vi "Read JsonContent.vi"(8 "error in (no error)":errorcluster, 11 "object in":refnum<class "TAFConfiguration.lvclass">) -> (0 "error out":errorcluster, 2 "JsonContent":string, 3 "object out":refnum<class "TAFConfiguration.lvclass">)   [LabVIEW 2021, in "TAF Proj Document Type.lvlib" / "TAFConfiguration.lvclass"]
uses:
  <vilib>/Wovalab/AntiDoc/Document Type/Add-ons/LabVIEW TAF Project/TAFConfiguration/TAFConfiguration.lvclass
  <vilib>/Wovalab/AntiDoc/Document Type/Add-ons/LabVIEW TAF Project/TAFConfiguration/TAFConfiguration.lvclass/TAFConfiguration.ctl
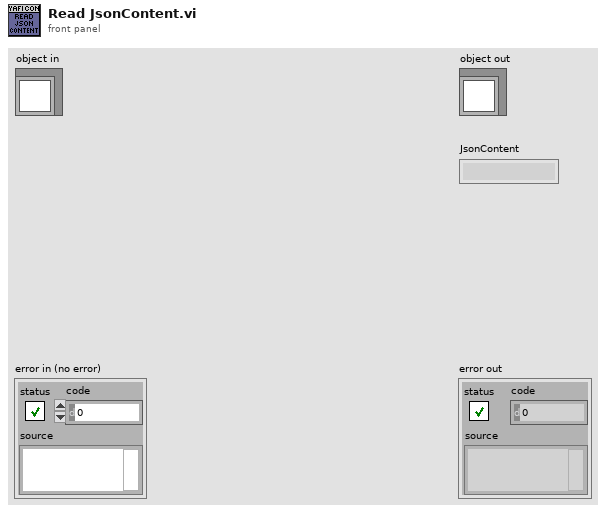
[diagram p1: front panel]
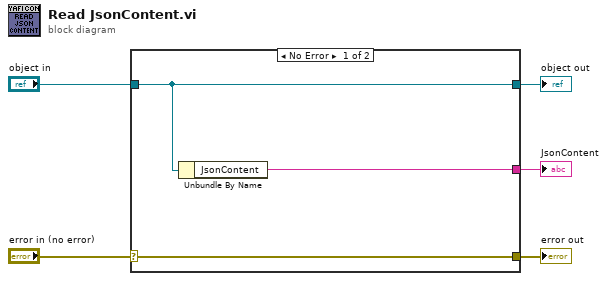
[diagram p0: block diagram]
diagram:
  n1 = case shown="No Error" "error in (no error)" {
    selector: "error in (no error)" -> [w8 w9]
    tunnel: [w8 w9] -> w4
    tunnel: [w7 w10] -> w2
    tunnel: "object in" -> [w7 w10]
    tunnel: [w6 _] -> w1
    frame No Error {
      n2 = Unbundle By Name(w7) -> ("JsonContent"=w6:string)
    }
    frame Error {
    }
  }
  "error out" <- w4
  "object out" <- w2
  "JsonContent" <- w1
